vi "BlinkM GetAddress.vi"(0 "Arduino Resource":T1={"VISA resource"="", "Board Type"=enum."Arduino Uno", "Connection Type"=enum."USB / Serial", "Bytes Per Packet (15)"=15}, 7 "Address":u8, 11 "error in":errorcluster) -> (4 "Arduino Resource":T1={"VISA resource"="", "Board Type"=enum."Arduino Uno", "Connection Type"=enum."USB / Serial", "Bytes Per Packet (15)"=15}, 8 "BlinkM Address":u8, 15 "error out":errorcluster)   [LabVIEW 2011, in "LabVIEW Interface for Arduino.lvlib"]
doc: "Get the address of the BlinkM. This VI can be used to determine the address of a single BlinkM on the I2C bus using the general call address (0x00)."
uses:
  LabVIEW Interface for Arduino.lvlib
  Private/Type Defs/Arduino Resource.ctl
  Private/Type Defs/Board Type.ctl
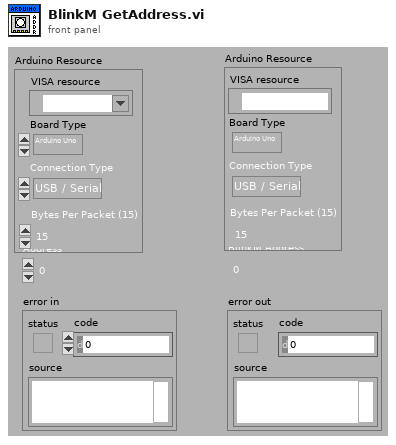
[diagram p1: front panel]
types:
  T1 = typedef "LabVIEW Interface for Arduino.lvlib/Arduino Resource.ctl" = cluster{"VISA resource":refnum<visa-resource-name>, "Board Type":T2, "Connection Type":enum8{"USB / Serial"}, "Bytes Per Packet (15)":u8}
  T2 = typedef "LabVIEW Interface for Arduino.lvlib/Board Type.ctl" = enum16{"Arduino Uno", "Dimuelanove w/Atmega 328", "Mega 2560", "Chipkit Uno32", "Chipkit Max32"}
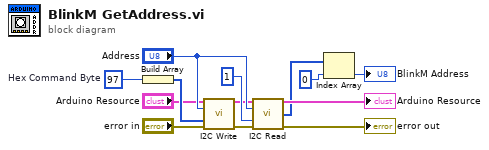
[diagram p0: block diagram]
diagram:
  w12 = u8 97  # Hex Command Byte
  n1 = Build Array(w12) -> (w11:u8[])
  n2 = call "I2C Write.vi"("Arduino Resource"="Arduino Resource", "Address (0)"="Address", "I2C Data Bytes"=w11, "error in"="error in") -> ("Arduino Resource"=w5:T1, "error out"=w10:errorcluster)  [unwired: 10 in]
  n3 = call "I2C Read.vi"("Arduino Resource"=w5, "Address (0)"="Address", "Bytes To Read"=u8 1, "error in"=w10) -> ("Arduino Resource"=→"Arduino Resource":T1, "I2C Data"=w2:u8[], "error out"=→"error out":errorcluster)  [unwired: 9 in]
  n4 = Index Array(array=w2, index=0) -> (element=→"BlinkM Address":u8)
